vi "Test Dummy API.vi"() -> ()   [LabVIEW 2020]
doc: "Dummy API Tester.\n\n____\nHAMPEL SOFTWARE ENGINEERING v2.6.0 (2023-12-19 10:54)"
uses:
  Libraries/hse-libraries/Source/hse-dqmh/Controls/Module Display Scenarios.ctl
  <vilib>/Utility/error.llb/DialogType.ctl
  <vilib>/Hampel Software Engineering/HSE Logger/LogRecord/LogRecord.lvclass/LogRecord.ctl
  Dummy.lvlib
  Libraries/hse-libraries/Source/hse-dqmh/hse-dqmh.lvlib
  <vilib>/Hampel Software Engineering/HSE Logger/hse-logger.lvlib
  <vilib>/Hampel Software Engineering/HSE Logger/LogRecord/LogRecord.lvclass
panel:
  in  "Show Main VI Diagram on Init (F)":bool
  in  "Request UI Display":bool
  in  "Prepare":bool
  in  "Configure":bool
  in  "Module Display Scenarios":T1
  in  "Show Block Diagram":bool
  in  "Stop Module":bool
  in  "Start Module":bool
  in  "Hide Module Panel":bool
  in  "Show Module Panel":bool
  out "Status":string
  out "Module Running?":bool
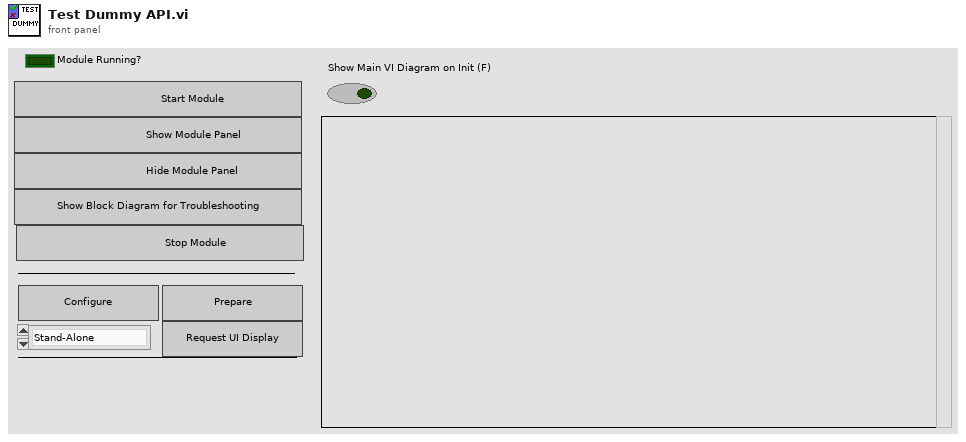
[diagram p1: front panel]
types:
  T1 = typedef "hse-dqmh.lvlib/Module Display Scenarios.ctl" = enum16{"Stand-Alone", "Managed"}
  T2 = typedef "Dummy.lvlib/Broadcast Events--cluster.ctl" = cluster{"Module Did Init":refnum<user-event>, "Status Updated":refnum<user-event>, "Error Reported":refnum<user-event>, "Module Did Stop":refnum<user-event>, "Update Module Execution Status":refnum<user-event>, "System Message":refnum<user-event>}
  T3 = typedef "DialogType.ctl" = u16
  T4 = typedef "hse-dqmh.lvlib/System Message Source.ctl" = enum16{"module", "application", "network"}
  T5 = typedef "hse-logger.lvlib/LogLevel.ctl" = enum16{"DEBUG", "INFO", "WARNING", "ERROR", "CRITICAL"}
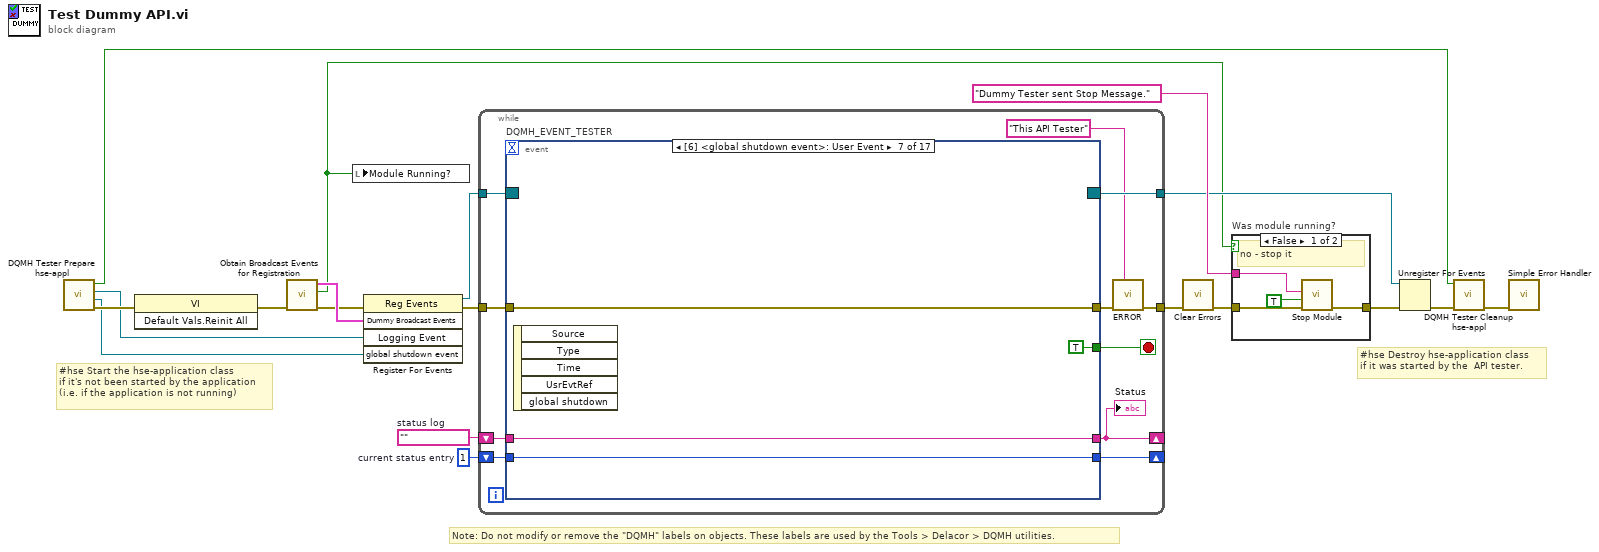
[diagram p0: block diagram]
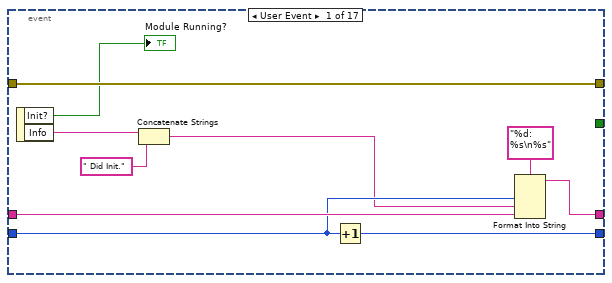
[diagram p3: hidden frame]
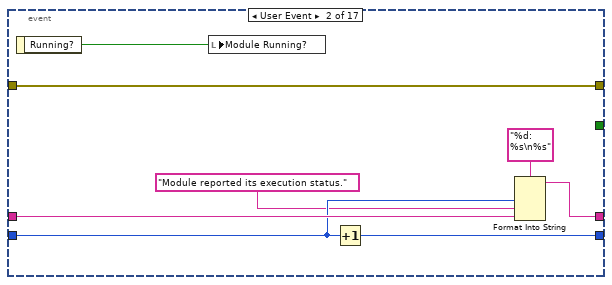
[diagram p4: hidden frame]
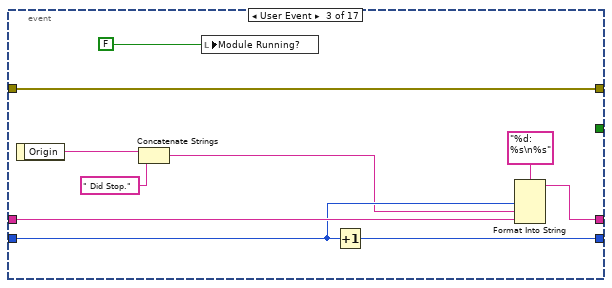
[diagram p5: hidden frame]
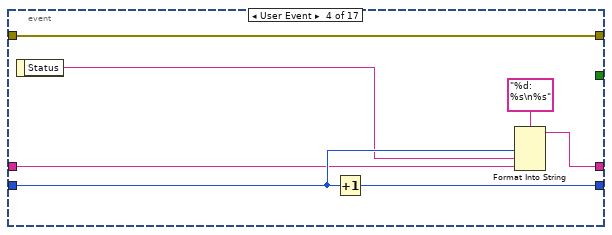
[diagram p6: hidden frame]
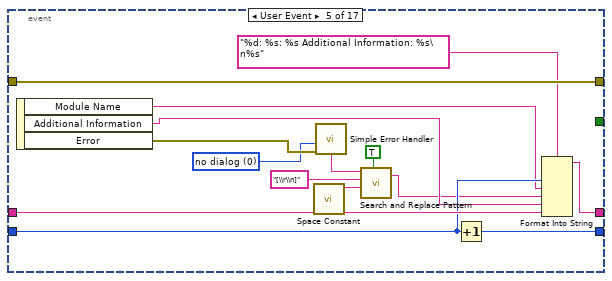
[diagram p7: hidden frame]
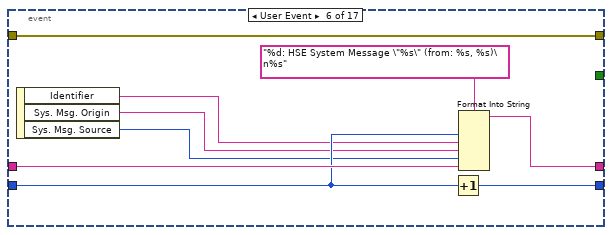
[diagram p8: hidden frame]
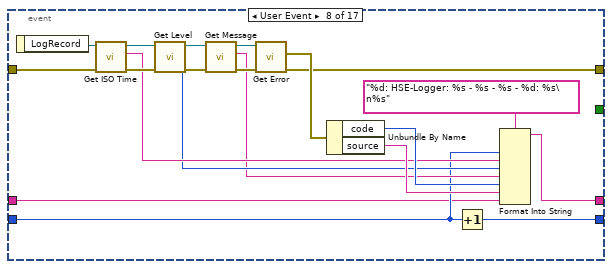
[diagram p9: hidden frame]
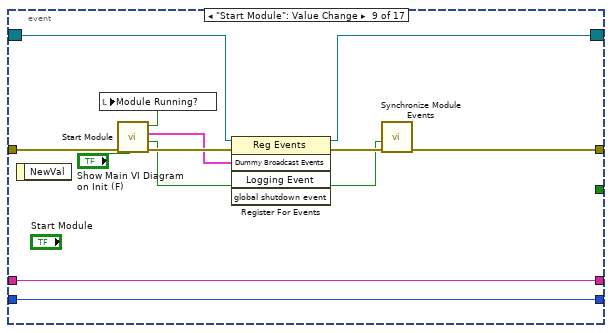
[diagram p10: hidden frame]
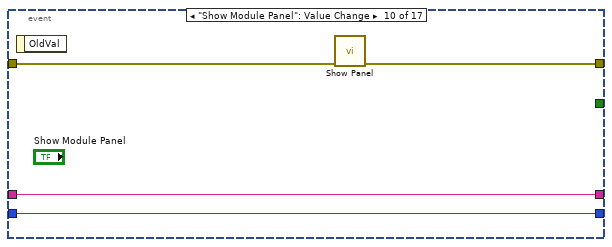
[diagram p11: hidden frame]
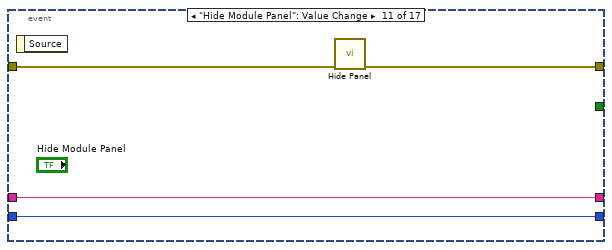
[diagram p12: hidden frame]
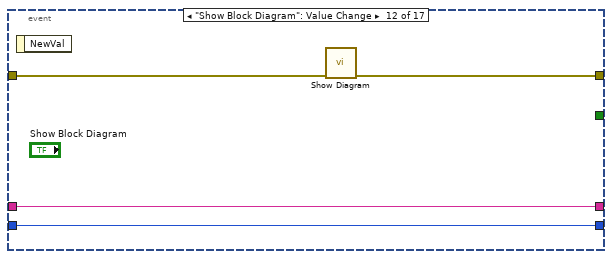
[diagram p13: hidden frame]
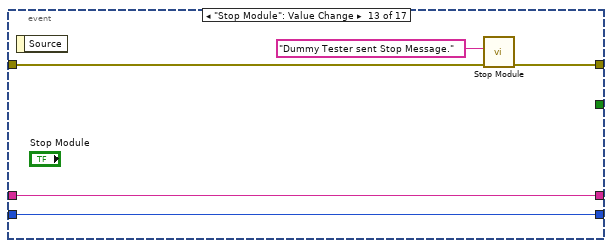
[diagram p14: hidden frame]
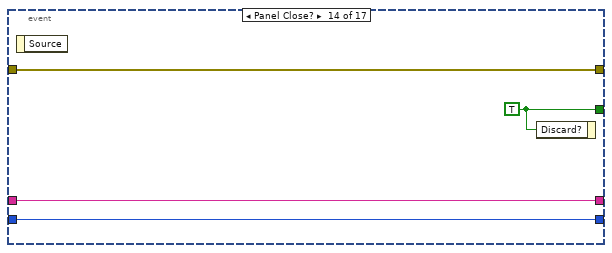
[diagram p15: hidden frame]
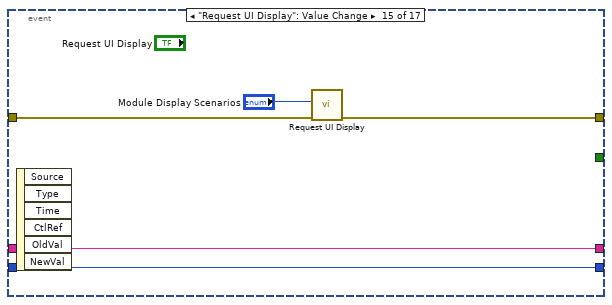
[diagram p16: hidden frame]
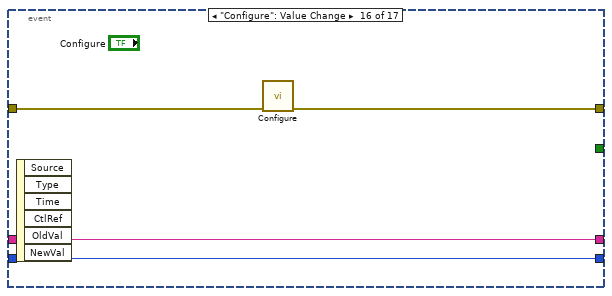
[diagram p17: hidden frame]
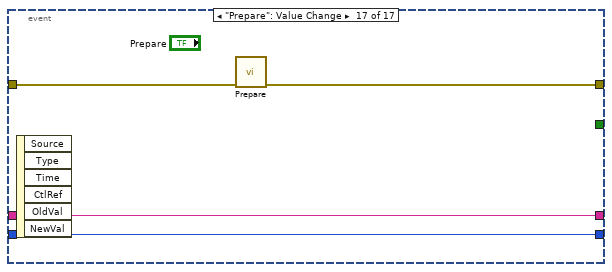
[diagram p18: hidden frame]
diagram:
  w16 = 1  # current status entry
  w17 = ""  # status log
  # "#hse Destroy hse-application class \nif it was started by the  API tester."
  # "#hse Start the hse-application class \nif it's not been started by the application\n(i.e. if the application is not running)"
  # "Note: Do not modify or remove the \"DQMH\" labels on objects. These labels are used by the Tools > Delacor > DQMH utilities."
  n1 = call "DQMH Tester Prepare hse-appl.vi"() -> ("error out"=w7:errorcluster, "global shutdown event"=w1:refnum<user-event>, "Logging Event"=w6:refnum<user-event>, "Started?"=w4:bool)  [unwired: 8 in]
  n2 = invoke class="VI" method="Default Vals.Reinit All"(error in=w7) -> (error out=w9:errorcluster)  [unwired: 2 in, 2 out]
  n3 = call "Obtain Broadcast Events for Registration.vi"("error in (no error)"=w9) -> ("error out"=w8:errorcluster, "Already running?"=w3:bool, "Dummy Broadcast Events"=w14:T2)  [unwired: 8 in]
  n4 = local write "Module Running?"(w3) -> ()
  n5 = register-events(error in=w8, w14, w6, w1) -> (reference out=w13:refnum<event-registration>, error out=w15:errorcluster)  [unwired: 1 in]
  n6 = while {
    tunnel: w13 -> [w30]
    tunnel: [w21] -> w10
    shift-right: [w26] -> _
    shift-left: w17 -> [w28]
    shift-right: [w27] -> _
    shift-left: w16 -> [w29]
    tunnel: w15 -> [w25]
    tunnel: [w24] -> w12
    stop <- w22 stop-if-true
    n7 = event "DQMH_EVENT_TESTER" shown="[6] <global shutdown event>: User Event" {
      selector: w30 -> [_ _ _ _ _ _ _ _ w119 _ _ _ _ _ _ _ _]
      dyn-events: [_ _ _ _ _ _ _ _ w118 _ _ _ _ _ _ _ _] -> w24
      timeout: _ -> [_ _ _ _ _ _ _ _ _ _ _ _ _ _ _ _ _]
      tunnel: [_ _ _ _ _ _ TRUE ("Discard?") _ _ _ _ _ _ w146 _ _ _] -> w22
      tunnel: [w40 w42 w49 w59 w80 w89 w93 w94 w117 w129 w133 w134 w140 w143 w148 w152 w156] -> w23
      tunnel: w29 -> [w36 w46 w56 w62 w77 w86 w91 w98 w122 w127 w131 w135 w141 w144 w149 w154 w158]
      tunnel: w28 -> [w37 w47 w57 w61 w79 w87 w92 w97 w123 w128 w132 w136 w142 w145 w150 w155 w159]
      tunnel: [w34 w44 w54 w63 w78 w85 w92 w100 w123 w128 w132 w136 w142 w145 w150 w155 w159] -> w26
      tunnel: [w35 w45 w55 w65 w76 w84 w91 w99 w122 w127 w131 w135 w141 w144 w149 w154 w158] -> w27
      tunnel: w25 -> [w40 w42 w49 w59 w80 w89 w93 w96 w116 w126 w130 w137 w138 w143 w151 w153 w157]
      event User Event {
        n8 = event-data() -> ("Init?"=→"Module Running?":bool, "Info"=w33:string)  [unwired: 1 in]
        n9 = Concatenate Strings(w33, " Did Init.") -> (w32:string)
        n10 = Increment(x=w36) -> (x+1=w35:i32)
        n11 = Format Into String(format string="%d: %s\n%s", w36, w32, w37) -> (resulting string=w34:string)  [unwired: 2 in, 1 out]
      }
      event User Event {
        n12 = event-data() -> ("Running?"=w41:bool)  [unwired: 1 in]
        n13 = local write "Module Running?"(w41) -> ()
        n14 = Increment(x=w46) -> (x+1=w45:i32)
        n15 = Format Into String(format string="%d: %s\n%s", w46, "Module reported its execution status.", w47) -> (resulting string=w44:string)  [unwired: 2 in, 1 out]
      }
      event User Event {
        n16 = event-data() -> ("Origin"=w53:string)  [unwired: 1 in]
        n17 = Concatenate Strings(w53, " Did Stop.") -> (w52:string)
        n18 = local write "Module Running?"(FALSE ("Module Did Init?")) -> ()
        n19 = Increment(x=w56) -> (x+1=w55:i32)
        n20 = Format Into String(format string="%d: %s\n%s", w56, w52, w57) -> (resulting string=w54:string)  [unwired: 2 in, 1 out]
      }
      event User Event {
        n21 = event-data() -> ("Status"=w60:string)  [unwired: 1 in]
        n22 = Increment(x=w62) -> (x+1=w65:i32)
        n23 = Format Into String(format string="%d: %s\n%s", w62, w60, w61) -> (resulting string=w63:string)  [unwired: 2 in, 1 out]
      }
      event User Event {
        w72 = T3 0 items=["no dialog", "OK message", "continue or stop message", "OK message + warnings", "continue/stop + warnings"] ("type of dialog (OK msg:1)")
        n24 = event-data() -> ("Module Name"=w73:string, "Additional Information"=w74:string, "Error"=w75:errorcluster)  [unwired: 1 in]
        n25 = call <vilib>:"Space Constant.vi"() -> ("String"=w68:string)
        n26 = call <vilib>:"Simple Error Handler.vi"("type of dialog (OK msg:1)"=w72, "error in (no error)"=w75) -> ("message"=w71:string)  [unwired: 3 in, 4 out]
        n27 = call <vilib>:"Search and Replace Pattern.vi"("string"=w71, "regular expression (\"\")"="[\\r\\n]" ("regular expression (\"\")"), "replace string (\"\")"=w68, "replace all? (F)"=TRUE ("replace all CR/LF with spaces")) -> ("result string"=w70:string)  [unwired: 1 in, 1 out]
        n28 = Increment(x=w77) -> (x+1=w76:i32)
        n29 = Format Into String(format string="%d: %s: %s Additional Information: %s\n%s", w77, w73, w70, w74, w79) -> (resulting string=w78:string)  [unwired: 2 in, 1 out]
      }
      event User Event {
        n30 = event-data() -> ("Identifier"=w83:string, "Sys. Msg. Origin"=w82:string, "Sys. Msg. Source"=w81:T4)  [unwired: 1 in]
        n31 = Increment(x=w86) -> (x+1=w84:i32)
        n32 = Format Into String(format string="%d: HSE System Message \"%s\" (from: %s, %s)\n%s", w86, w83, w82, w81, w87) -> (resulting string=w85:string)  [unwired: 2 in, 1 out]
      }
      event User Event {
        n33 = event-data() -> ()  [unwired: 1 in, 5 out]
      }
      event User Event {
        n34 = event-data() -> ("LogRecord"=w95:refnum<class "LogRecord.lvclass">)  [unwired: 1 in]
        n35 = call <vilib>:"Get ISO Time.vi"("error in"=w96, "LogRecord in"=w95) -> ("error out"=w113:errorcluster, "ISO Time"=w104:string, "LogRecord out"=w110:refnum<class "LogRecord.lvclass">)  [unwired: 7 in]
        n36 = call <vilib>:"Get Level.vi"("error in"=w113, "LogRecord in"=w110) -> ("error out"=w112:errorcluster, "Level"=w103:T5, "LogRecord out"=w109:refnum<class "LogRecord.lvclass">)  [unwired: 7 in]
        n37 = call <vilib>:"Get Message.vi"("error in"=w112, "LogRecord in"=w109) -> ("error out"=w111:errorcluster, "Message"=w102:string, "LogRecord out"=w108:refnum<class "LogRecord.lvclass">)  [unwired: 7 in]
        n38 = call <vilib>:"Get Error.vi"("error in"=w111, "LogRecord in"=w108) -> ("error out"=w94:errorcluster, "Error"=w105:errorcluster)  [unwired: 7 in, 1 out]
        n39 = Unbundle By Name(w105) -> ("code"=w106:i32, "source"=w107:string)
        n40 = Increment(x=w98) -> (x+1=w99:i32)
        n41 = Format Into String(format string="%d: HSE-Logger: %s - %s - %s - %d: %s\n%s", w98, w104, w103, w102, w106, w107, w97) -> (resulting string=w100:string)  [unwired: 2 in, 1 out]
      }
      event "Start Module": Value Change {
        n42 = event-data() -> ()  [unwired: 1 in, 1 out]
        n43 = call "Start Module.vi"("Show Main VI Diagram on Init (F)"="Show Main VI Diagram on Init (F)", "error in (no error)"=w116) -> ("error out"=w124:errorcluster, "Wait for Event Sync?"=w121:bool, "Dummy Broadcast Events"=w120:T2, "Module Was Already Running?"=w115:bool)  [unwired: 6 in]
        n44 = local write "Module Running?"(w115) -> ()
        n45 = register-events(reference=w119, error in=w124, w120) -> (reference out=w118:refnum<event-registration>, error out=w125:errorcluster)  [unwired: 2 in]
        n46 = call "Synchronize Module Events.vi"("error in (no error)"=w125, "Wait for Event Sync?"=w121) -> ("error out"=w117:errorcluster)  [unwired: 9 in]
      }
      event "Show Module Panel": Value Change {
        n47 = event-data() -> ()  [unwired: 1 in, 1 out]
        n48 = call "Show Panel.vi"("error in (no error)"=w126) -> ("error out"=w129:errorcluster)  [unwired: 10 in]
      }
      event "Hide Module Panel": Value Change {
        n49 = event-data() -> ()  [unwired: 1 in, 1 out]
        n50 = call "Hide Panel.vi"("error in (no error)"=w130) -> ("error out"=w133:errorcluster)  [unwired: 10 in]
      }
      event "Show Block Diagram": Value Change {
        n51 = event-data() -> ()  [unwired: 1 in, 1 out]
        n52 = call "Show Diagram.vi"("error in (no error)"=w137) -> ("error out"=w134:errorcluster)  [unwired: 10 in]
      }
      event "Stop Module": Value Change {
        n53 = event-data() -> ()  [unwired: 1 in, 1 out]
        n54 = call "Stop Module.vi"("error in (no error)"=w138, "Origin"="Dummy Tester sent Stop Message.") -> ("error out"=w140:errorcluster)  [unwired: 9 in]
      }
      event Panel Close? {
        w146 = TRUE ("Discard?")
        n55 = event-data() -> ()  [unwired: 1 in, 1 out]
        n56 = event-data("Discard?"=w146) -> ()  [unwired: 1 in, 1 out]
      }
      event "Request UI Display": Value Change {
        n57 = event-data() -> ()  [unwired: 1 in, 6 out]
        n58 = call "Request UI Display.vi"("error in (no error)"=w151, "Scenario"="Module Display Scenarios") -> ("error out"=w148:errorcluster)  [unwired: 8 in, 1 out]
      }
      event "Configure": Value Change {
        n59 = event-data() -> ()  [unwired: 1 in, 6 out]
        n60 = call "Configure.vi"("error in (no error)"=w153) -> ("error out"=w152:errorcluster)  [unwired: 10 in]
      }
      event "Prepare": Value Change {
        n61 = event-data() -> ()  [unwired: 1 in, 6 out]
        n62 = call "Prepare.vi"("error in (no error)"=w157) -> ("error out"=w156:errorcluster)  [unwired: 10 in]
      }
    }
    "Status" <- w26
    n63 = call <vilib>:"ERROR.vi"("Message"="This API Tester" ("Origin"), "error in"=w23) -> ("error out"=w21:errorcluster)  [unwired: 9 in]
  }
  n64 = call <vilib>:"Clear Errors.vi"("error in (no error)"=w10) -> ("error out"=w11:errorcluster)  [unwired: 5 in, 1 out]
  n65 = case "Was module running?" shown="False" w3 {
    tunnel: [w163 w164] -> w19
    tunnel: "Dummy Tester sent Stop Message." ("Origin") -> [w162 _]
    tunnel: w11 -> [w160 w164]
    frame False {
      # "no - stop it"
      n66 = call "Stop Module.vi"("error in (no error)"=w160, "Wait for Module to Stop? (F)"=TRUE ("Wait for Module to stop?"), "Origin"=w162) -> ("error out"=w163:errorcluster)  [unwired: 8 in]
    }
    frame True {
      # "yes - do nothing"
    }
  }
  n67 = Unregister For Events(event registration refnum=w12, error in=w19) -> (error out=w5:errorcluster)
  n68 = call "DQMH Tester Cleanup hse-appl.vi"("error in"=w5, "Stop?"=w4) -> ("error out"=w2:errorcluster)  [unwired: 9 in]
  n69 = call <vilib>:"Simple Error Handler.vi"("error in (no error)"=w2) -> ()  [unwired: 4 in, 5 out]
